vi "Helium Fridge Cool-Down-old.vi"() -> ()   [LabVIEW 2014]
uses:
  <vilib>/Analysis/8numeric.llb/1D Numeric Integration.vi
  <vilib>/express/express shared/transition.llb/Dynamic To Waveform Array.vi
  <vilib>/express/express signal manip/GetorSetDDTAttributes/Set DDT Attributes/SetT0.vi
  <vilib>/express/express shared/transition.llb/Waveform Array To Dynamic.vi
  <vilib>/express/express signal manip/GetorSetDDTAttributes/Set DDT Attributes/Set DDT Properties.xnode
  <vilib>/Analysis/NI_AALPro.lvlib
panel:
  out "?":dbl
  out "?":dbl
  out "?":dbl
  out "?":dbl
  out "Baseline X":dbl[](array[numeric])
  out "Session Out 2":refnum<visa-resource-name>
  out "error out 2":errorcluster {"code" format="%.0x"}
  out "token":dbl
  in  "error in 2":errorcluster {"code" format="%.0x"}
  in  "Session In 2":refnum<visa-resource-name>="HPSIGGEN"
  in  "Depth/Div Submit":bool
  out "Depth/Div (kHz)":dbl
  in  "Cent. Frq. Submit":bool
  out "Session Out":refnum<visa-resource-name>
  out "error out":errorcluster {"code" format="%.0x"}
  out "Central Frequency":dbl
  in  "error in":errorcluster {"code" format="%.0x"}
  in  "Session In":refnum<visa-resource-name>="HPSIGGEN"
  out "Cent. Freq. (MHz)":dbl
  out "Temp 2":bool
  out "Temperature Strip Chart":dynamicdata(graph)
  in  "TC Points/Measurement":dbl=20.0
  out "NMR":bool
  out "NMR Temp Error":bool
  out "Q Meter Temp":dynamicdata(graph)
  out "Zeroed Array":dbl[](array[numeric])
  out "Fit X values":dbl[](array[numeric])
  in  "Left wing 2":dbl
  in  "Right wing 2":dbl
  in  "Right wing":dbl
  in  "Left wing":dbl
  out "Fit":dbl[](array[numeric])
  in  "Submit":bool
  out "Is Flashing":bool
  in  "Error Beat":bool
  in  "Clear":bool
  in  "Comment":string
  out "Heartbeat":bool
  out "Most Recent Error":string
  out "Baseline Subtracted Integral vs. Time":dbl(graph)
  out "Time of Last Baseline":string
  out "Baseline Y":dbl[](array[numeric])
  in  "Baseline Subtract":bool
  in  "Get Baseline":bool
  out "Recording":bool
  out "Time of Last Recording":string
  in  "Record \nNMR Sweeps":bool
  in  "Depth/Div\n(MHz)":dbl=0.5
  in  "Central Freq. \n(MHz)":dbl=12.996
  in  "stop (F)":bool caption="Triangle Wave"
  in  "Triangle Wave\nRate (Hz)":dbl=15.0
  out "Time Elapsed \nDuring Sweeps (s)":dbl
  out "Lab Time":string
  out "Most Recent Error (NMR)":string
  out "Last Sweep Start Time":string
  out "Most Recent Error (Temp)":string
  out "Last Measurement Taken":string
  out "VI Start Time":string
  in  "Time Between\nTemp Ponts (s)":dbl=5.0
  out "Temp":bool
  out "NMR":bool
  in  "stop":bool
  out "Input Triangle Wave":dynamicdata(graph)
  out "Modulator":dynamicdata(graph)
  out "NMR":cluster{"Y":dbl[], "Y":dbl[]}[](graph)
  in  "# of Sweeps":dbl=1.0
  out "Resistance Strip Chart":dynamicdata(graph)
  in  "Heartbeat":bool
  in  "Temp Strip Chart":bool
  out "Errors":bool
  in  "Silence Flashing":bool
  # "Signal Generator Logic -- DO NOT TOUCH!!"
  # "Initialization and Logic Controls -- DO NOT TOUCH!!"
  # "Caitlyn's Work"
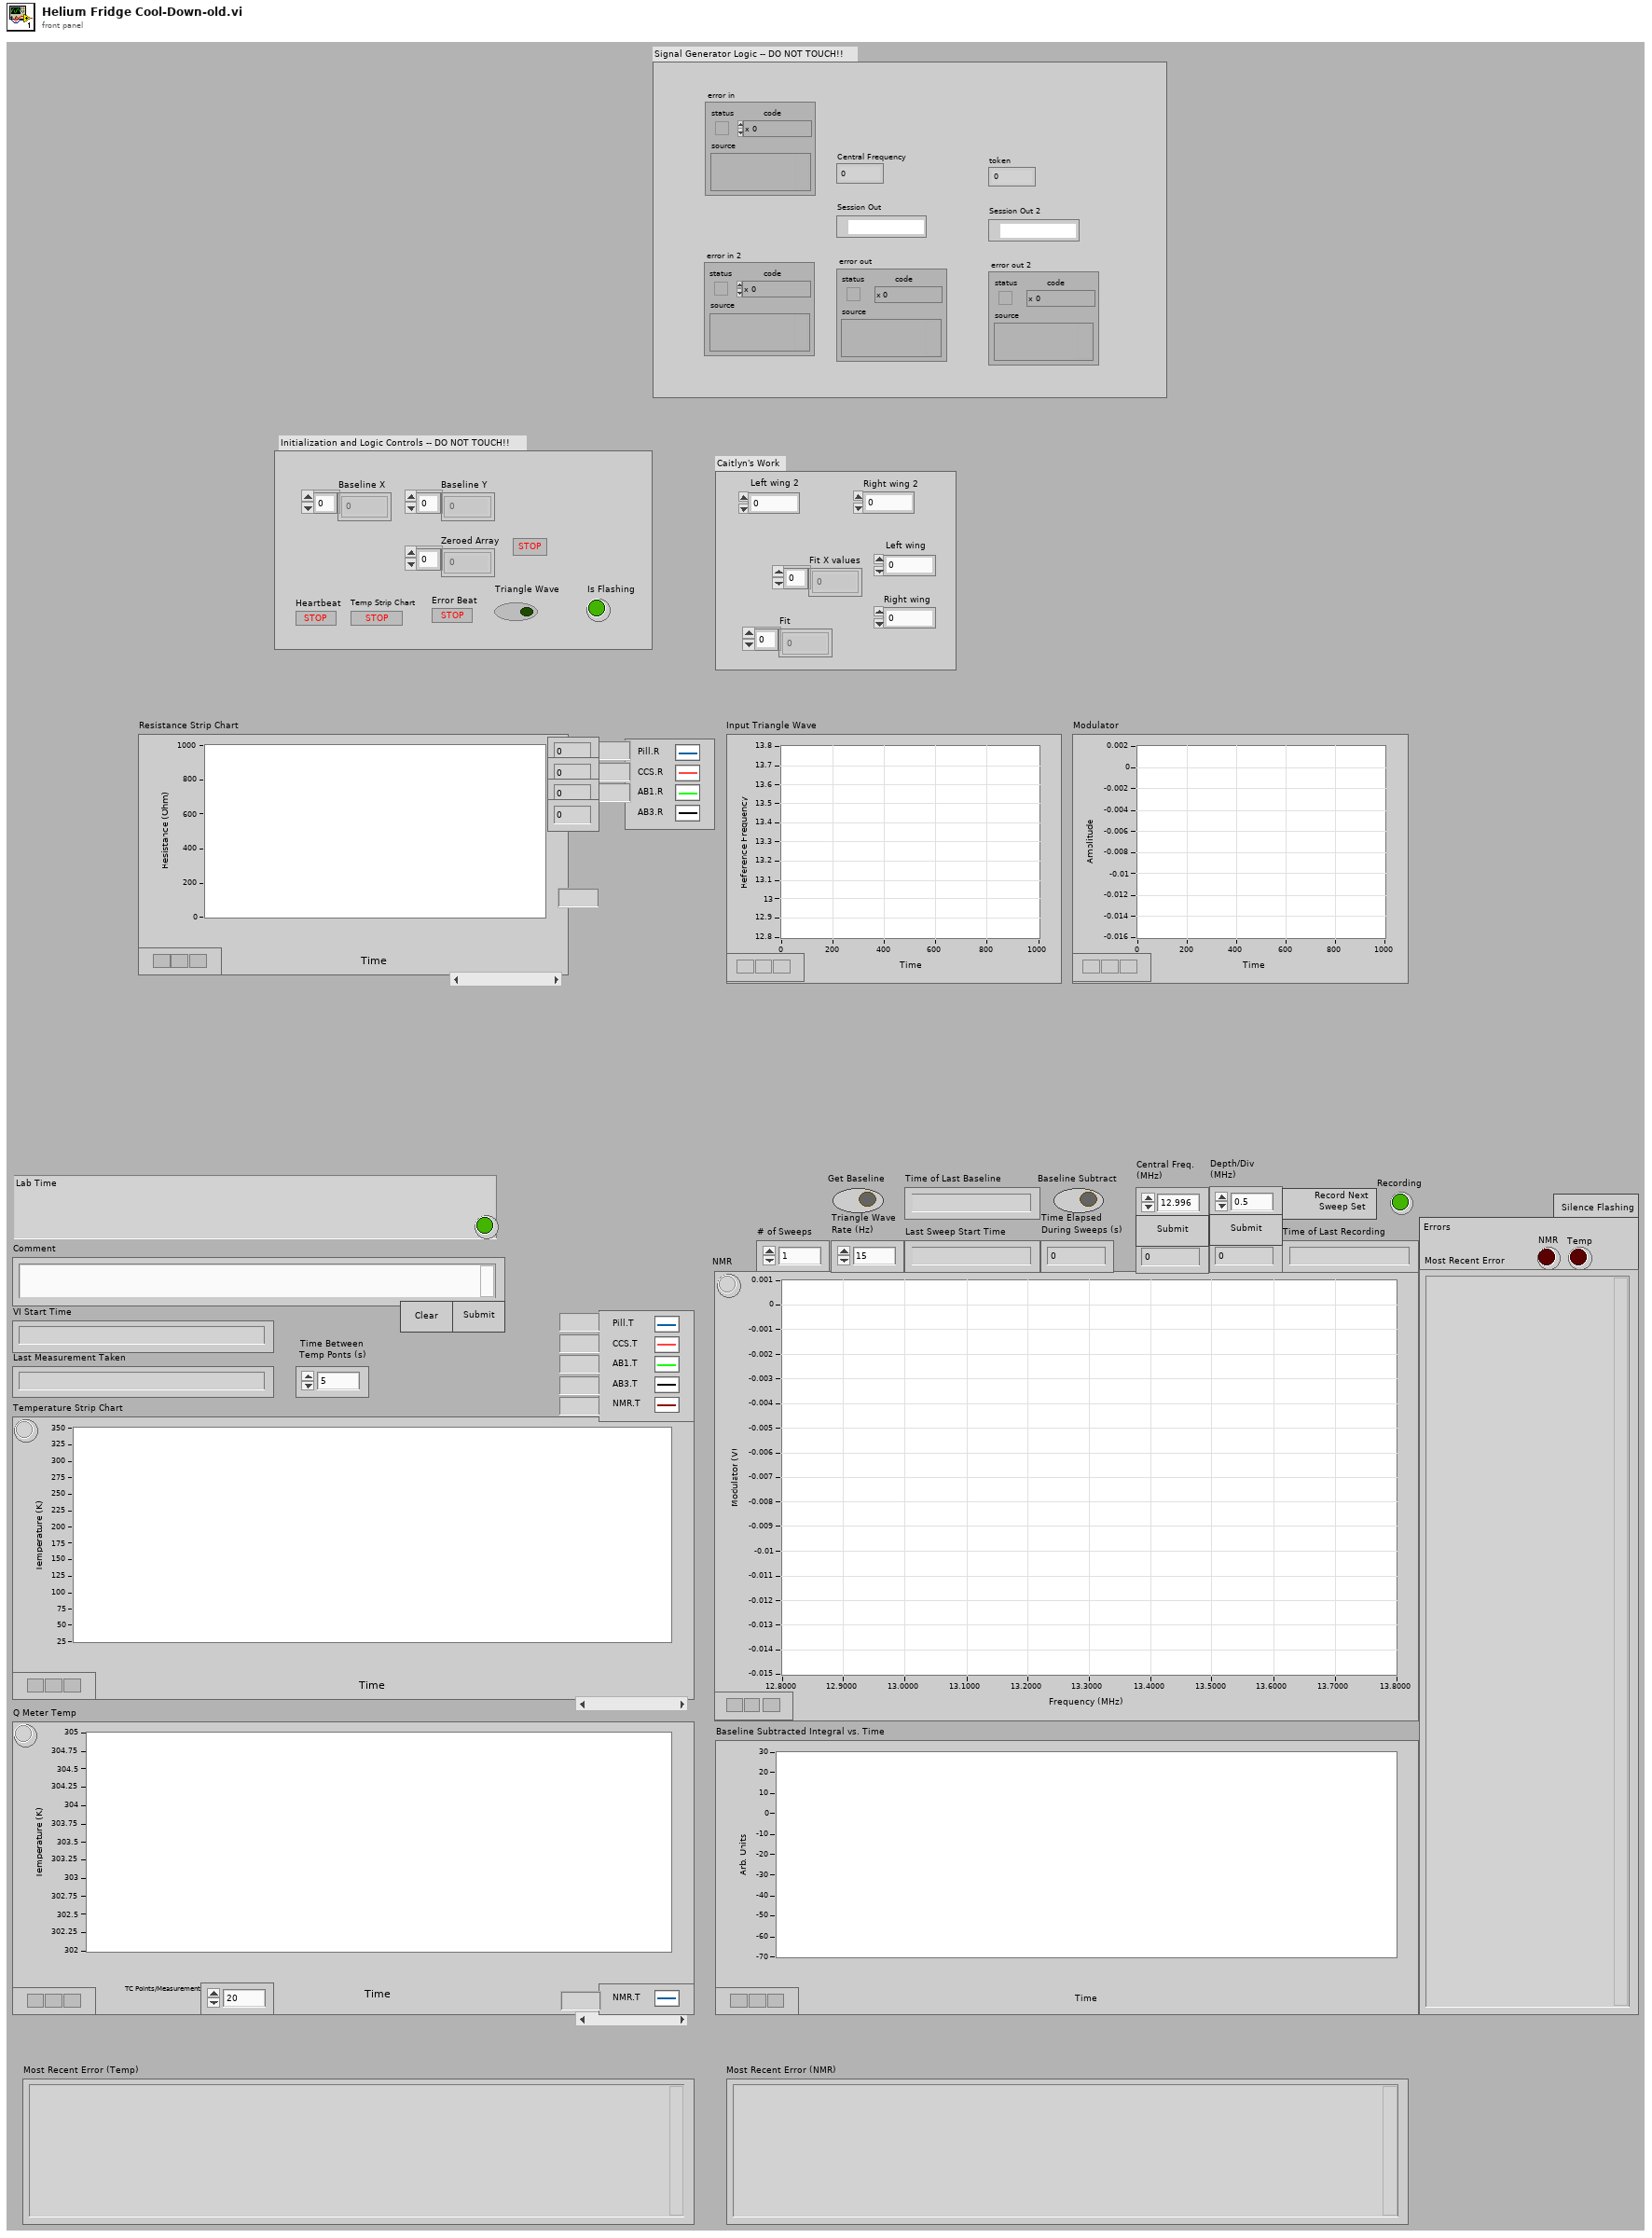
[diagram p1: front panel]
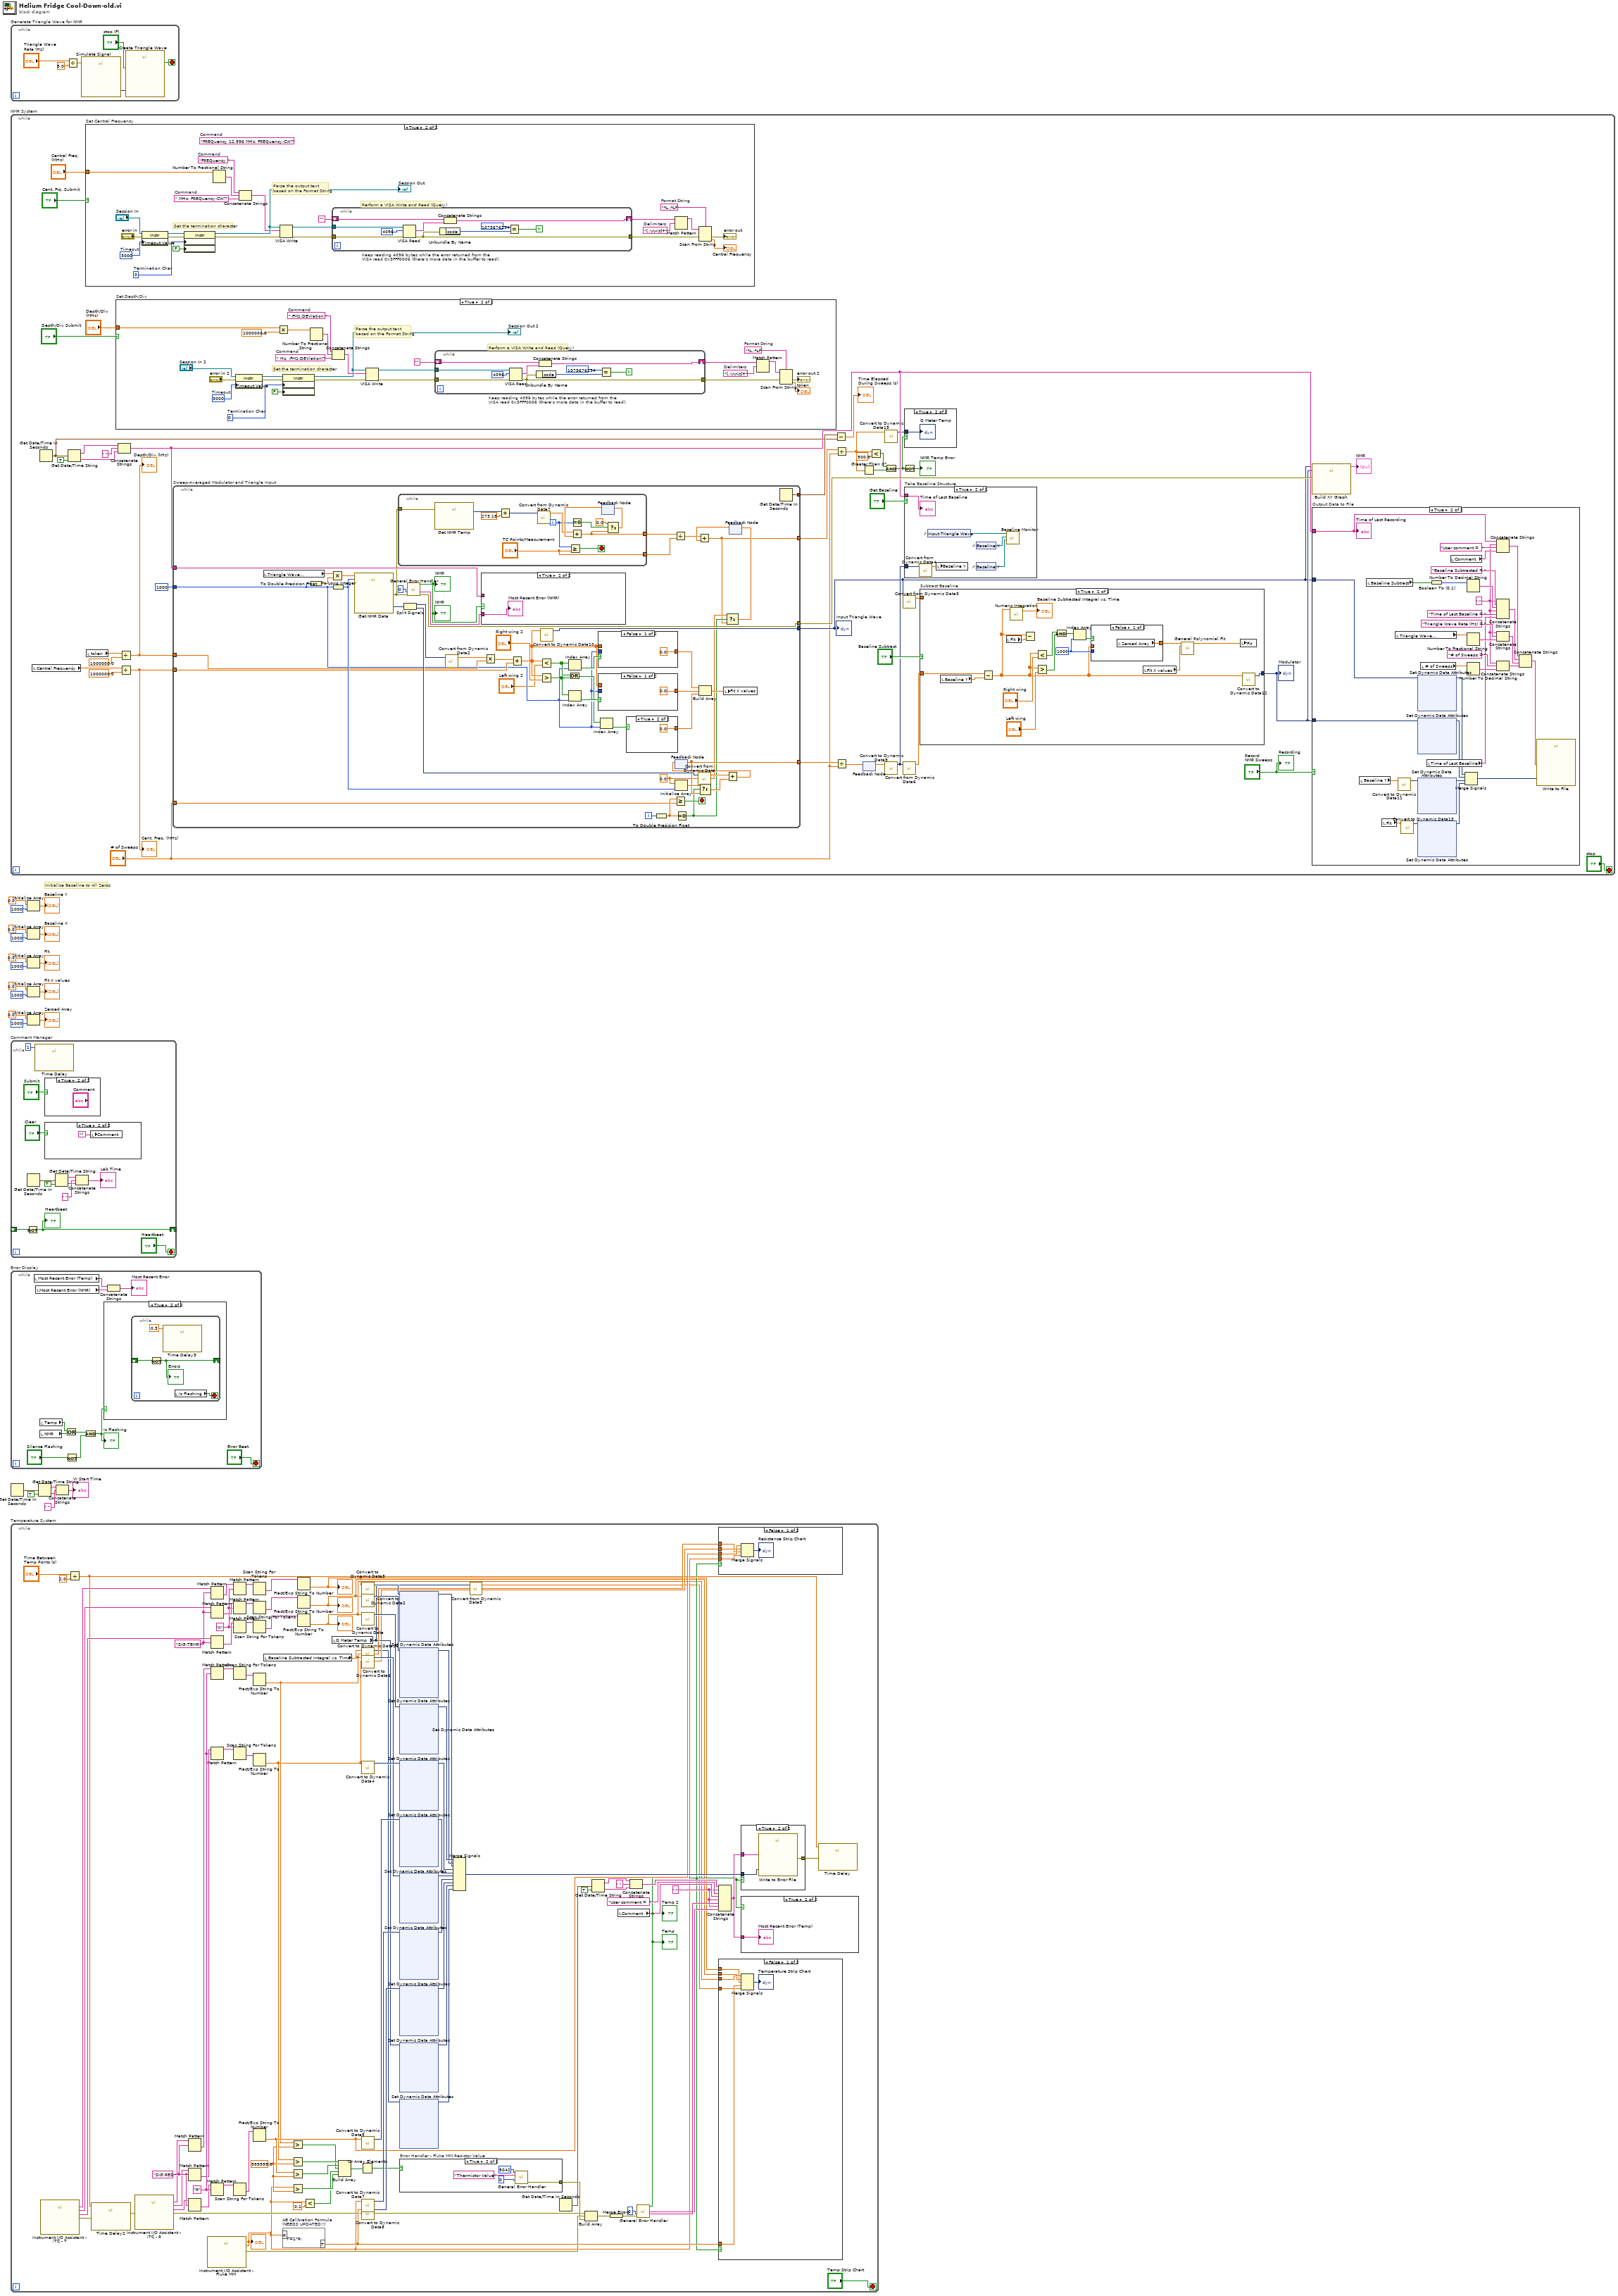
[diagram p0: block diagram]
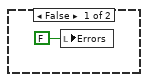
[diagram p2: hidden frame]
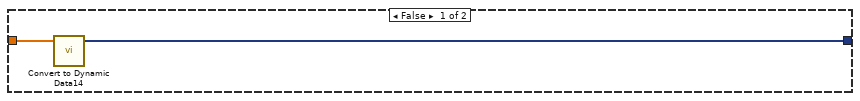
[diagram p6: hidden frame]
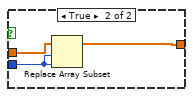
[diagram p7: hidden frame]
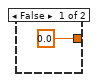
[diagram p10: hidden frame]
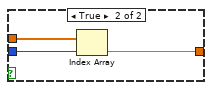
[diagram p11: hidden frame]
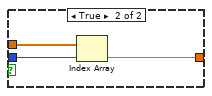
[diagram p12: hidden frame]
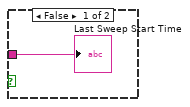
[diagram p13: hidden frame]
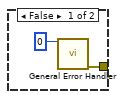
[diagram p16: hidden frame]
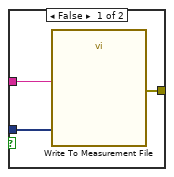
[diagram p19: hidden frame]
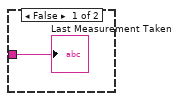
[diagram p20: hidden frame]
diagram:
  # "Initialize Baseline to All Zeros"
  n1 = while "Generate Triangle Wave for NMR" {
    stop <- w26 stop-if-true
    n2 = Divide(x="Triangle Wave\nRate (Hz)", y=5.0) -> (x/y=w22:dbl)
    n3 = call "Simulate Signal"("Frequency"=w22) -> ("Triangle"=w25:dynamicdata)  [unwired: 13 in, 1 out]
    n4 = call "Create Triangle Wave"("data"=w25, "stop (F)"="stop (F)") -> ("stopped"=w26:bool)  [unwired: 15 in, 2 out]
  }
  n5 = while "NMR System" {
    stop <- "stop" stop-if-true
    n6 = local read "Central Frequency"() -> (w34:dbl)
    n7 = Get Date/Time In Seconds() -> (seconds since 1Jan1904=w58:timestamp)
    n8 = Get Date/Time String(seconds (now)=w58, want seconds? (F)=TRUE) -> (date string=w61:string, time string=w63:string)  [unwired: 1 in]
    n9 = case "Set Central Frequency" shown="True" "Cent. Frq. Submit" {
      tunnel: "Central Freq. \n(MHz)" -> [_ w109]
      frame False {
      }
      frame True {
        w107 = " MHz; FREQuency:CW?"  # Command
        w110 = "FREQuency "  # Command
        w128 = "[,;\r\n\t]+"  # Delimiters
        w125 = "%.;%f"  # Format String
        (unwired) "FREQuency 12.996 MHz; FREQuency:CW?"  # Command
        w116 = u8 0  # Termination Char
        w111 = u32 3000  # Timeout
        # "Parse the output text based on the Format String"
        # "Perform a VISA Write and Read (Query)"
        # "Keep reading 4096 bytes while the error returned from the\nVISA read 0x3FFF0006 (there's more data in the buffer to read)."
        # "Set the termination character"
        n10 = property class="Instr"(reference="Session In", error in="error in", "General Settings:Timeout Value"=w111) -> (reference out=w117:refnum<visa-resource-name>, error out=w114:errorcluster)
        n11 = property class="Instr"(reference=w117, error in=w114, "Message Based Settings:Termination Character"=w116, "Message Based Settings:Termination Character Enable"=FALSE ("enable")) -> (reference out=w129:refnum<visa-resource-name>, error out=w115:errorcluster)
        "Session Out" <- w129
        n12 = Number To Fractional String(number=w109) -> (F-format string=w108:string)  [unwired: 3 in]
        n13 = Concatenate Strings(w110, w108, w107) -> (w106:string)
        n14 = VISA Write(VISA resource name=w129, write buffer=w106, error in (no error)=w115) -> (VISA resource name out=w119:refnum<visa-resource-name>, error out=w120:errorcluster)  [unwired: 1 out]
        n15 = while {
          tunnel: w119 -> [w136]
          shift-right: [w130] -> w123
          shift-left: "" -> [w135]
          tunnel: w120 -> [w133]
          tunnel: [w132] -> w121
          stop <- w131 continue-if-true
          n16 = VISA Read(VISA resource name=w136, byte count=u32 4096 ("byte count (0)"), error in (no error)=w133) -> (read buffer=w134:string, error out=w132:errorcluster)  [unwired: 2 out]
          n17 = Unbundle By Name(w132) -> ("code"=w138:i32)
          n18 = Concatenate Strings(w135, w134) -> (w130:string)
          n19 = Equal?(x=1073676294, y=w138) -> (x = y?=w131:bool)
        }
        n20 = Match Pattern(string=w123, regular expression=w128) -> (before substring=w124:string)  [unwired: 1 in, 3 out]
        n21 = Scan From String(format string=w125, input string=w124, error in=w121) -> (error out=→"error out":errorcluster, output 1=→"Central Frequency":dbl)  [unwired: 2 in, 2 out]
      }
    }
    n22 = local read "token"() -> (w29:dbl)
    n23 = case "Set Depth/Div" shown="True" "Depth/Div Submit" {
      tunnel: "Depth/Div\n(MHz)" -> [_ w71]
      frame False {
      }
      frame True {
        w73 = " Hz; :FM1:DEViation?"  # Command
        w78 = "[,;\r\n\t]+"  # Delimiters
        w81 = "%.;%f"  # Format String
        w75 = ":FM1:DEViation "  # Command
        w90 = u8 0  # Termination Char
        w95 = u32 3000  # Timeout
        # "Parse the output text based on the Format String"
        # "Perform a VISA Write and Read (Query)"
        # "Keep reading 4096 bytes while the error returned from the\nVISA read 0x3FFF0006 (there's more data in the buffer to read)."
        # "Set the termination character"
        n24 = property class="Instr"(reference="Session In 2", error in="error in 2", "General Settings:Timeout Value"=w95) -> (reference out=w89:refnum<visa-resource-name>, error out=w92:errorcluster)
        n25 = Multiply(x=w71, y=1000000.0) -> (x*y=w70:dbl)
        n26 = property class="Instr"(reference=w89, error in=w92, "Message Based Settings:Termination Character"=w90, "Message Based Settings:Termination Character Enable"=FALSE ("enable")) -> (reference out=w77:refnum<visa-resource-name>, error out=w91:errorcluster)
        "Session Out 2" <- w77
        n27 = Number To Fractional String(number=w70) -> (F-format string=w74:string)  [unwired: 3 in]
        n28 = Concatenate Strings(w75, w74, w73) -> (w76:string)
        n29 = VISA Write(VISA resource name=w77, write buffer=w76, error in (no error)=w91) -> (VISA resource name out=w87:refnum<visa-resource-name>, error out=w86:errorcluster)  [unwired: 1 out]
        n30 = while {
          tunnel: w87 -> [w102]
          shift-right: [w96] -> w83
          shift-left: "" -> [w101]
          tunnel: w86 -> [w99]
          tunnel: [w98] -> w85
          stop <- w97 continue-if-true
          n31 = VISA Read(VISA resource name=w102, byte count=u32 4096 ("byte count (0)"), error in (no error)=w99) -> (read buffer=w100:string, error out=w98:errorcluster)  [unwired: 2 out]
          n32 = Unbundle By Name(w98) -> ("code"=w104:i32)
          n33 = Concatenate Strings(w101, w100) -> (w96:string)
          n34 = Equal?(x=1073676294, y=w104) -> (x = y?=w97:bool)
        }
        n35 = Match Pattern(string=w83, regular expression=w78) -> (before substring=w82:string)  [unwired: 1 in, 3 out]
        n36 = Scan From String(format string=w81, input string=w82, error in=w85) -> (error out=→"error out 2":errorcluster, output 1=→"token":dbl)  [unwired: 2 in, 2 out]
      }
    }
    n37 = Concatenate Strings(w61, " ", w63) -> (w49:string)
    n38 = Divide(x=w29, y=1000000.0) -> (x/y=w28:dbl)
    "Depth/Div (kHz)" <- w28
    n39 = Divide(x=w34, y=1000000.0) -> (x/y=w32:dbl)
    "Cent. Freq. (MHz)" <- w32
    n40 = while "Sweep-Averaged Modulator and Triangle Input" {
      tunnel: "# of Sweeps" -> [w297]
      tunnel: 1000 -> [w288]
      tunnel: [w314] -> w66
      tunnel: w49 -> [w310]
      tunnel: [w309] -> w59
      tunnel: [w307] -> w56
      tunnel: w28 -> [w301]
      tunnel: w32 -> [w299]
      tunnel: [w298] -> w48
      tunnel: [w278] -> w37
      i -> [w320]
      stop <- w313 stop-if-true
      w281 = 0.0
      n41 = local read "Triangle Wave\nRate (Hz)"() -> (w306:dbl)
      n42 = To Double Precision Float(number=w288) -> (double precision float=w304:dbl)
      n43 = Multiply(x=w306, y=w304) -> (x*y=w308:dbl)
      n44 = To Long Integer(number=w288) -> (32bit integer=w305:i32)
      n45 = call "Get NMR Data"("rate"=w308, "number of samples"=w305) -> ("data"=w322:dynamicdata, "error out"=w273:errorcluster)  [unwired: 15 in, 1 out]
      n46 = while {
        tunnel: ["TC Points/Measurement"] -> w276
        tunnel: [w327] -> w275
        tunnel: w273 -> [w326]
        i -> [w325]
        stop <- w324 stop-if-true
        n47 = call "Get NMR Temp"("error in"=w326) -> ("data"=w329:dynamicdata)  [unwired: 16 in, 2 out]
        n48 = Add(x=w329, y=273.15) -> (x+y=w328:dynamicdata)
        n49 = call "Convert from Dynamic Data7"("Dynamic Data Type"=w328) -> ("Scalar"=w331:dbl)  [unwired: 3 in]
        n50 = Greater Or Equal?(x=w325, y="TC Points/Measurement") -> (x >= y?=w324:bool)
        n51 = Equal To 0?(x=w325) -> (x = 0?=w332:bool)
        n52 = feedback #1() -> (w334:dbl)  [unwired: 1 in]
        n53 = Add(x=w331, y=w334) -> (x+y=w327:dbl)
        n54 = Select(t=0.0, s=w332, f=w327) -> (s? t:f=w333:dbl)
        n55 = feedback-in #1(w333) -> ()
      }
      n56 = Split Signals(w322) -> (w303:dynamicdata, w321:dynamicdata)  [unwired: 2 in]
      n57 = call <vilib>:"General Error Handler.vi"("type of dialog (OK msg:1)"=0, "error in (no error)"=w273) -> ("error?"=w277:bool, "message"=w312:string, "error out"=w307:errorcluster)  [unwired: 9 in, 2 out]
      "NMR" <- w277
      "NMR" <- w277
      n58 = call "Convert from Dynamic Data2"("Dynamic Data Type"=w303) -> ("Array"=w302:dbl[])  [unwired: 3 in]
      n59 = case shown="True" w277 {
        tunnel: w312 -> [_ w347]
        tunnel: w310 -> [w346 _]
        frame False {
          "Last Sweep Start Time" <- w346
        }
        frame True {
          "Most Recent Error (NMR)" <- w347
        }
      }
      n60 = Multiply(x=w302, y=w301) -> (x*y=w300:dbl[])
      n61 = Add(x=w300, y=w299) -> (x+y=w294:dbl[])
      n62 = Less?(x=w294, y="Left wing 2") -> (x < y?=w290:bool[])
      n63 = Greater?(x=w294, y="Right wing 2") -> (0:w291:bool[])
      n64 = call "Convert to Dynamic Data10"("Array"=w294) -> ("Dynamic Data Type"=w298:dynamicdata)  [unwired: 3 in]
      n65 = Or(x=w290, y=w291) -> (x .or. y?=w289:bool[])
      n66 = Index Array(array=w290, index=w288) -> (element=w296:bool)
      n67 = Index Array(array=w291, index=w288) -> (element=w295:bool)
      n68 = case shown="False" w296 {
        tunnel: w294 -> [_ w345]
        tunnel: w288 -> [_ w344]
        tunnel: [0.0 w343] -> w292
        frame False {
        }
        frame True {
          n69 = Index Array(array=w345, index=w344) -> (element=w343:dbl)
        }
      }
      n70 = case shown="False" w295 {
        tunnel: w294 -> [_ w341]
        tunnel: w288 -> [_ w340]
        tunnel: [0.0 w339] -> w293
        frame False {
        }
        frame True {
          n71 = Index Array(array=w341, index=w340) -> (element=w339:dbl)
        }
      }
      n72 = Index Array(array=w289, index=w288) -> (element=w287:bool)
      n73 = case shown="True" w287 {
        tunnel: [0.0 0.0] -> w286
        frame False {
        }
        frame True {
        }
      }
      n74 = To Double Precision Float(number=w320) -> (double precision float=w319:dbl)
      n75 = Divide(x=w275, y=w276) -> (x/y=w274:dbl)
      n76 = Greater Or Equal?(x=w319, y=w297) -> (x >= y?=w313:bool)
      n77 = feedback #2() -> (w314:dbl[])  [unwired: 1 in]
      n78 = Initialize Array(w281, w305) -> (w317:dbl[])
      n79 = Equal To 0?(x=w319) -> (x = 0?=w282:bool)
      n80 = call "Convert from Dynamic Data"("Dynamic Data Type"=w321) -> ("Array"=w316:dbl[])  [unwired: 3 in]
      n81 = Build Array(w292, w293, w286) -> (w283:dbl[])
      n82 = Select(t=w317, s=w282, f=w314) -> (s? t:f=w318:dbl[])
      n83 = local write "Fit X values"(w283) -> ()
      n84 = Add(x=w316, y=w318) -> (x+y=w315:dbl[])
      n85 = feedback-in #2(w315) -> ()
      n86 = feedback #3() -> (w279:dbl)  [unwired: 1 in]
      n87 = Add(x=w274, y=w279) -> (x+y=w278:dbl)
      n88 = Select(t=w281, s=w282, f=w278) -> (s? t:f=w280:dbl)
      n89 = feedback-in #3(w280) -> ()
      n90 = Get Date/Time In Seconds() -> (seconds since 1Jan1904=w309:timestamp)
    }
    "Input Triangle Wave" <- w48
    n91 = Subtract(x=w59, y=w58) -> (x-y=→"Time Elapsed \nDuring Sweeps (s)":dbl)
    n92 = Divide(x=w37, y="# of Sweeps") -> (x/y=w38:dbl)
    n93 = Divide(x=w66, y="# of Sweeps") -> (x/y=w65:dbl[])
    n94 = Greater Than 0?(x=w38) -> (x > 0?=w45:bool)
    n95 = feedback-in #4(w65) -> ()
    n96 = feedback #4() -> (w64:dbl[])  [unwired: 1 in]
    n97 = Less?(x=w38, y=500.0) -> (x < y?=w42:bool)
    n98 = call "Convert to Dynamic Data15"("Double"=w38) -> ("Dynamic Data Type"=w40:dynamicdata)  [unwired: 3 in]
    n99 = And(x=w42, y=w45) -> (x .and. y?=w44:bool)
    n100 = call "Convert to Dynamic Data9"("Array"=w64) -> ("Dynamic Data Type"=w51:dynamicdata)  [unwired: 3 in]
    n101 = Not(x=w44) -> (.not. x?=→"NMR Temp Error":bool)
    n102 = call "Convert from Dynamic Data3"("Dynamic Data Type"=w48) -> ("Array"=w47:dbl[])  [unwired: 3 in]
    n103 = call "Convert from Dynamic Data6"("Dynamic Data Type"=w51) -> ("Array"=w46:dbl[])  [unwired: 3 in]
    n104 = case shown="True" w44 {
      tunnel: w40 -> [_ w140]
      frame False {
      }
      frame True {
        "Q Meter Temp" <- w140
      }
    }
    n105 = case "Take Baseline Structure" shown="True" "Get Baseline" {
      tunnel: w51 -> [_ w166]
      tunnel: w49 -> [_ w167]
      frame False {
      }
      frame True {
        n106 = call "Convert from Dynamic Data4"("Dynamic Data Type"=w166) -> ("Array"=w168:dbl[])  [unwired: 3 in]
        n107 = control-ref of="Input Triangle Wave"() -> (w165:refnum<vi>)
        n108 = local write "Baseline Y"(w168) -> ()
        n109 = control-ref of="Baseline X"() -> (w164:refnum<vi>)
        n110 = control-ref of="Baseline Y"() -> (w163:refnum<vi>)
        n111 = call "Baseline Monitor.vi"("reference 3"=w163, "reference in"=w164, "WaveformGraph in"=w165) -> ()  [unwired: 8 in, 1 out]
        "Time of Last Baseline" <- w167
      }
    }
    n112 = case "Subtract Baseline" shown="True" "Baseline Subtract" {
      tunnel: w46 -> [w142 w158]
      tunnel: [w141 w157] -> w50
      tunnel: w47 -> [_ _]
      frame False {
        n113 = call "Convert to Dynamic Data14"("Array"=w142) -> ("Dynamic Data Type"=w141:dynamicdata)  [unwired: 3 in]
      }
      frame True {
        w147 = 1000
        n114 = local read "Baseline Y"() -> (w155:dbl[])
        n115 = Subtract(x=w158, y=w155) -> (x-y=w143:dbl[])
        n116 = local read "Fit"() -> (w154:dbl[])
        n117 = call-poly <vilib>:"Numeric Integration.vi"("Input Array"=w143) -> ("result"=→"Baseline Subtracted Integral vs. Time":dbl)  [unwired: 2 in, 1 out]
        n118 = Subtract(x=w143, y=w154) -> ()  [unwired: 1 out]
        n119 = Less?(x=w143, y="Right wing") -> (x < y?=w151:bool[])
        n120 = Greater?(x=w143, y="Left wing") -> (0:w150:bool[])
        n121 = And(x=w151, y=w150) -> (x .and. y?=w149:bool[])
        n122 = Index Array(array=w149, index=w147) -> (element=w148:bool)
        n123 = case shown="False" w148 {
          tunnel: w143 -> [_ w162]
          tunnel: w147 -> [_ w160]
          tunnel: [w159 w161] -> w146
          frame False {
            n124 = local read "Zeroed Array"() -> (w159:dbl[])
          }
          frame True {
            n125 = Replace Array Subset(array=w162, new element=w160, index=w160) -> (w161:dbl[])
          }
        }
        n126 = local read "Fit X values"() -> (w144:dbl[])
        n127 = call <vilib>:"General Polynomial Fit.vi"("Y"=w146, "X"=w144) -> ("Best Polynomial Fit"=w145:dbl[])  [unwired: 10 in, 3 out]
        n128 = local write "Fit"(w145) -> ()
        n129 = call "Convert to Dynamic Data12"("Array"=w143) -> ("Dynamic Data Type"=w157:dynamicdata)  [unwired: 3 in]
      }
    }
    "Modulator" <- w50
    n130 = call "Build XY Graph"("error in (no error)"=w56, "Y Input"=w50, "X Input"=w48) -> ("XY Graph"=→"NMR":cluster{"Y":dbl[], "Y":dbl[]}[])  [unwired: 7 in, 1 out]
    n131 = case "Output Data to File" shown="True" "Record \nNMR Sweeps" {
      tunnel: w49 -> [_ w189]
      tunnel: w50 -> [_ w196]
      tunnel: w48 -> [_ w195]
      frame False {
      }
      frame True {
        w173 = ";"
        n132 = local read "Baseline Y"() -> (w194:dbl[])
        n133 = local read "Baseline Subtract"() -> (w191:bool)
        n134 = local read "Fit"() -> (w172:dbl[])
        n135 = local read "Triangle Wave\nRate (Hz)"() -> (w192:dbl)
        n136 = call "Convert to Dynamic Data11"("Array"=w194) -> ("Dynamic Data Type"=w193:dynamicdata)  [unwired: 3 in]
        n137 = call "Convert to Dynamic Data13"("Array"=w172) -> ("Dynamic Data Type"=w171:dynamicdata)  [unwired: 3 in]
        n138 = xnode "Set Dynamic Data Attributes"("Signals In"=w195) -> ("Signals Out"=w200:dynamicdata)  [unwired: 4 in, 1 out]
        n139 = xnode "Set Dynamic Data Attributes"("Signals In"=w196) -> ("Signals Out"=w198:dynamicdata)  [unwired: 4 in, 1 out]
        n140 = xnode "Set Dynamic Data Attributes"("Signals In"=w193) -> ("Signals Out"=w170:dynamicdata)  [unwired: 4 in, 1 out]
        n141 = xnode "Set Dynamic Data Attributes"("Signals In"=w171) -> ("Signals Out"=w169:dynamicdata)  [unwired: 4 in, 1 out]
        n142 = local read "# of Sweeps"() -> (w197:dbl)
        n143 = local read "Time of Last Baseline"() -> (w178:string)
        n144 = Boolean To (0,1)(Boolean=w191) -> (0, 1=w190:i16)
        n145 = local read "Comment"() -> (w187:string)
        n146 = Merge Signals(w200, w198, w170, w169) -> (w199:dynamicdata)
        n147 = Number To Decimal String(number=w190) -> (decimal integer string=w183:string)  [unwired: 1 in]
        n148 = Number To Fractional String(number=w192) -> (F-format string=w181:string)  [unwired: 3 in]
        n149 = Number To Decimal String(number=w197) -> (decimal integer string=w185:string)  [unwired: 1 in]
        n150 = Concatenate Strings(w189, w173, "User comment =  ", w187) -> (w180:string)
        n151 = Concatenate Strings(w173, "Baseline Subtracted = ", w183, w173, "Time of Last Baseline = ", w178) -> (w177:string)
        n152 = Concatenate Strings(w173, "Triangle Wave Rate (Hz) = ", w181) -> (w176:string)
        n153 = Concatenate Strings(w173, "# of Sweeps = ", w185) -> (w175:string)
        n154 = Concatenate Strings(w180, w177, w176, w175) -> (w174:string)
        n155 = call "Write to File"("Signals"=w199, "Comment"=w174) -> ()  [unwired: 15 in, 3 out]
        "Time of Last Recording" <- w189
      }
    }
    "Recording" <- "Record \nNMR Sweeps"
  }
  n156 = while "Comment Manager" {
    shift-right: [w356] -> _
    shift-left: _ -> [w359]
    stop <- "Heartbeat" stop-if-true
    n157 = Not(x=w359) -> (.not. x?=w356:bool)
    "Heartbeat" <- w356
    n158 = Get Date/Time In Seconds() -> (seconds since 1Jan1904=w354:timestamp)
    n159 = call "Time Delay"("Delay Time (s)"=1) -> ()  [unwired: 10 in, 1 out]
    n160 = case shown="True" "Submit" {
      frame False {
      }
      frame True {
      }
    }
    n161 = case shown="True" "Clear" {
      frame False {
      }
      frame True {
        n162 = local write "Comment"("") -> ()
      }
    }
    n163 = Get Date/Time String(seconds (now)=w354, want seconds? (F)=TRUE) -> (date string=w353:string, time string=w351:string)  [unwired: 1 in]
    n164 = Concatenate Strings(w353, " ", w351) -> (→"Lab Time":string)
  }
  n165 = while "Error Display" {
    stop <- "Error Beat" stop-if-true
    n166 = local read "Most Recent Error (Temp)"() -> (w361:string)
    n167 = local read "Most Recent Error (NMR)"() -> (w362:string)
    n168 = local read "Temp"() -> (w370:bool)
    n169 = local read "NMR"() -> (w369:bool)
    n170 = Or(x=w370, y=w369) -> (x .or. y?=w367:bool)
    n171 = Not(x="Silence Flashing") -> (.not. x?=w365:bool)
    n172 = And(x=w367, y=w365) -> (x .and. y?=w364:bool)
    "Is Flashing" <- w364
    n173 = case shown="True" w364 {
      frame False {
        n174 = local write "Errors"(FALSE) -> ()
      }
      frame True {
        n175 = while {
          shift-right: [w373] -> _
          shift-left: _ -> [w375]
          stop <- w372 stop-if-true
          n176 = Not(x=w375) -> (.not. x?=w373:bool)
          "Errors" <- w373
          n177 = call "Time Delay3"("Delay Time (s)"=0.3) -> ()  [unwired: 10 in, 1 out]
          n178 = local read "Is Flashing"() -> (w372:bool)
        }
      }
    }
    n179 = Concatenate Strings(w361, w362) -> (→"Most Recent Error":string)
  }
  n180 = Get Date/Time In Seconds() -> (seconds since 1Jan1904=w20:timestamp)
  n181 = while "Temperature System" {
    stop <- "Temp Strip Chart" stop-if-true
    w389 = ";"
    w410 = 999999.0
    w439 = "R"
    w440 = "SIG:RES:"
    w446 = "SIG:TEMP:"
    w445 = "K"
    n182 = call "Instrument I/O Assistant - iTC - T"() -> ("AB1.T"=w444:string, "CCS.T"=w449:string, "Pill.T"=w452:string, "error out"=w402:errorcluster)  [unwired: 23 in, 1 out]
    n183 = Divide(x="Time Between\nTemp Ponts (s)", y=2.0) -> (x/y=w397:dbl)
    n184 = call "Time Delay2"("error in (no error)"=w402, "Delay Time (s)"=w397) -> ("error out"=w403:errorcluster)  [unwired: 9 in]
    n185 = call "Instrument I/O Assistant - iTC - R"("error in"=w403) -> ("AB1.R"=w399:string, "CCS.R"=w400:string, "Pill.R"=w401:string, "error out"=w404:errorcluster)  [unwired: 22 in, 1 out]
    n186 = Match Pattern(string=w399, regular expression=w440) -> (after substring=w436:string)  [unwired: 1 in, 3 out]
    n187 = Match Pattern(string=w400, regular expression=w440) -> (after substring=w438:string)  [unwired: 1 in, 3 out]
    n188 = Match Pattern(string=w401, regular expression=w440) -> (after substring=w437:string)  [unwired: 1 in, 3 out]
    n189 = call "Instrument I/O Assistant - Fluke MM"() -> ("AB3.R"=w379:dbl, "error out"=w407:errorcluster)  [unwired: 25 in, 1 out]
    "?" <- w379
    n190 = Match Pattern(string=w444, regular expression=w446) -> (after substring=w443:string)  [unwired: 1 in, 3 out]
    n191 = Match Pattern(string=w449, regular expression=w446) -> (after substring=w448:string)  [unwired: 1 in, 3 out]
    n192 = Match Pattern(string=w452, regular expression=w446) -> (after substring=w451:string)  [unwired: 1 in, 3 out]
    n193 = Match Pattern(string=w436, regular expression=w439) -> (before substring=w433:string)  [unwired: 1 in, 3 out]
    n194 = Match Pattern(string=w438, regular expression=w439) -> (before substring=w435:string)  [unwired: 1 in, 3 out]
    n195 = Match Pattern(string=w437, regular expression=w439) -> (before substring=w434:string)  [unwired: 1 in, 3 out]
    n196 = Match Pattern(string=w443, regular expression=w445) -> (before substring=w442:string)  [unwired: 1 in, 3 out]
    n197 = Match Pattern(string=w448, regular expression=w445) -> (before substring=w447:string)  [unwired: 1 in, 3 out]
    n198 = Match Pattern(string=w451, regular expression=w445) -> (before substring=w450:string)  [unwired: 1 in, 3 out]
    n199 = Scan String For Tokens(9:w433) -> (1:w430:string)  [unwired: 5 in, 3 out]
    n200 = Scan String For Tokens(9:w435) -> (1:w432:string)  [unwired: 5 in, 3 out]
    n201 = Scan String For Tokens(9:w434) -> (1:w431:string)  [unwired: 5 in, 3 out]
    n202 = Scan String For Tokens(9:w442) -> (1:w466:string)  [unwired: 5 in, 3 out]
    n203 = Scan String For Tokens(9:w447) -> (1:w467:string)  [unwired: 5 in, 3 out]
    n204 = Scan String For Tokens(9:w450) -> (1:w469:string)  [unwired: 5 in, 3 out]
    n205 = Fract/Exp String To Number(string=w430) -> (number=w414:dbl)  [unwired: 3 in, 1 out]
    n206 = Fract/Exp String To Number(string=w432) -> (number=w383:dbl)  [unwired: 3 in, 1 out]
    n207 = Fract/Exp String To Number(string=w431) -> (number=w415:dbl)  [unwired: 3 in, 1 out]
    n208 = local read "Baseline Subtracted Integral vs. Time"() -> (w378:dbl)
    n209 = formula code="T=1*R;" "AB Calibration Formula\n(NEEDS UPDATED!!)"("R"=w379) -> ("T"=w420:dbl)
    n210 = Greater?(x=w414, y=w410) -> (0:w411:bool)
    n211 = Greater?(x=w383, y=w410) -> (0:w413:bool)
    n212 = Greater?(x=w415, y=w410) -> (0:w412:bool)
    n213 = Greater?(x=w379, y=w410) -> (0:w409:bool)
    n214 = Fract/Exp String To Number(string=w466) -> (number=w380:dbl)  [unwired: 3 in, 1 out]
    "?" <- w380
    n215 = Fract/Exp String To Number(string=w467) -> (number=w381:dbl)  [unwired: 3 in, 1 out]
    "?" <- w381
    n216 = Fract/Exp String To Number(string=w469) -> (number=w382:dbl)  [unwired: 3 in, 1 out]
    "?" <- w382
    n217 = Less?(x=w379, y=0.1) -> (x < y?=w408:bool)
    n218 = local read "Q Meter Temp"() -> (w385:dynamicdata)
    n219 = Build Array(w413, w412, w411, w408, w409) -> (w417:bool[])
    n220 = Or Array Elements(Boolean array=w417) -> (logical OR=w416:bool)
    n221 = call "Convert to Dynamic Data3"("Double"=w380) -> ("Dynamic Data Type"=w457:dynamicdata)  [unwired: 3 in]
    n222 = call "Convert to Dynamic Data2"("Double"=w381) -> ("Dynamic Data Type"=w458:dynamicdata)  [unwired: 3 in]
    n223 = call "Convert to Dynamic Data"("Double"=w382) -> ("Dynamic Data Type"=w460:dynamicdata)  [unwired: 3 in]
    n224 = call "Convert to Dynamic Data16"("Double"=w378) -> ("Dynamic Data Type"=w377:dynamicdata)  [unwired: 3 in]
    n225 = call "Convert to Dynamic Data6"("Double"=w414) -> ("Dynamic Data Type"=w427:dynamicdata)  [unwired: 3 in]
    n226 = call "Convert to Dynamic Data4"("Double"=w383) -> ("Dynamic Data Type"=w429:dynamicdata)  [unwired: 3 in]
    n227 = call "Convert to Dynamic Data5"("Double"=w415) -> ("Dynamic Data Type"=w428:dynamicdata)  [unwired: 3 in]
    n228 = call "Convert to Dynamic Data7"("Double"=w379) -> ("Dynamic Data Type"=w423:dynamicdata)  [unwired: 3 in]
    n229 = call "Convert to Dynamic Data8"("Double"=w420) -> ("Dynamic Data Type"=w419:dynamicdata)  [unwired: 3 in]
    n230 = xnode "Set Dynamic Data Attributes"("Signals In"=w457) -> ("Signals Out"=w455:dynamicdata)  [unwired: 4 in, 1 out]
    n231 = xnode "Set Dynamic Data Attributes"("Signals In"=w458) -> ("Signals Out"=w456:dynamicdata)  [unwired: 4 in, 1 out]
    n232 = xnode "Set Dynamic Data Attributes"("Signals In"=w460) -> ("Signals Out"=w459:dynamicdata)  [unwired: 4 in, 1 out]
    n233 = xnode "Set Dynamic Data Attributes"("Signals In"=w429) -> ("Signals Out"=w426:dynamicdata)  [unwired: 4 in, 1 out]
    n234 = xnode "Set Dynamic Data Attributes"("Signals In"=w428) -> ("Signals Out"=w425:dynamicdata)  [unwired: 4 in, 1 out]
    n235 = xnode "Set Dynamic Data Attributes"("Signals In"=w427) -> ("Signals Out"=w424:dynamicdata)  [unwired: 4 in, 1 out]
    n236 = xnode "Set Dynamic Data Attributes"("Signals In"=w423) -> ("Signals Out"=w422:dynamicdata)  [unwired: 4 in, 1 out]
    n237 = xnode "Set Dynamic Data Attributes"("Signals In"=w419) -> ("Signals Out"=w418:dynamicdata)  [unwired: 4 in, 1 out]
    n238 = xnode "Set Dynamic Data Attributes"("Signals In"=w385) -> ("Signals Out"=w388:dynamicdata)  [unwired: 4 in, 1 out]
    n239 = xnode "Set Dynamic Data Attributes"("Signals In"=w377) -> ("Signals Out"=w376:dynamicdata)  [unwired: 4 in, 1 out]
    n240 = case "Error Handler - Fluke MM Resistor Value" shown="True" w416 {
      tunnel: [w506 w511] -> w406
      frame False {
        n241 = call <vilib>:"General Error Handler.vi"("[error code] (0)"=0) -> ("error out"=w506:errorcluster)  [unwired: 10 in, 4 out]
      }
      frame True {
        n242 = call <vilib>:"General Error Handler.vi"("[error code] (0)"=5042, "[error source] (\" \")"="Thermistor Value", "type of dialog (OK msg:1)"=0) -> ("error out"=w511:errorcluster)  [unwired: 8 in, 4 out]
      }
    }
    n243 = Merge Signals(w459, w456, w455, w426, w425, w424, w422, w418, w388, w376) -> (w454:dynamicdata)
    n244 = call "Convert from Dynamic Data5"("Dynamic Data Type"=w385) -> ("Scalar"=w384:dbl)  [unwired: 3 in]
    n245 = Get Date/Time In Seconds() -> (seconds since 1Jan1904=w465:timestamp)
    n246 = Build Array(w404, w407, w406) -> (w405:errorcluster[])
    n247 = Get Date/Time String(seconds (now)=w465, want seconds? (F)=TRUE) -> (date string=w463:string, time string=w461:string)  [unwired: 1 in]
    n248 = Merge Errors(w405) -> (w421:errorcluster)
    n249 = local read "Comment"() -> (w394:string)
    n250 = Concatenate Strings(w463, " ", w461) -> (w390:string)
    n251 = call <vilib>:"General Error Handler.vi"("type of dialog (OK msg:1)"=0, "error in (no error)"=w421) -> ("error?"=w386:bool, "source out"=w391:string, "message"=w393:string)  [unwired: 9 in, 2 out]
    "Temp" <- w386
    "Temp 2" <- w386
    n252 = case shown="False" w386 {
      tunnel: w415 -> [w606 _]
      tunnel: w383 -> [w605 _]
      tunnel: w414 -> [w604 _]
      tunnel: w379 -> [w603 _]
      frame False {
        n253 = Merge Signals(w606, w605, w604, w603) -> (→"Resistance Strip Chart":dynamicdata)
      }
      frame True {
      }
    }
    n254 = Concatenate Strings(w390, w389, "User comment =  ", w394, w389, w393, w389, w391) -> (w392:string)
    n255 = case shown="False" w386 {
      tunnel: w382 -> [w612 _]
      tunnel: w381 -> [w611 _]
      tunnel: w380 -> [w610 _]
      tunnel: w420 -> [w609 _]
      tunnel: w384 -> [w607 _]
      frame False {
        n256 = Merge Signals(w612, w611, w610, w609, w607) -> (→"Temperature Strip Chart":dynamicdata)
      }
      frame True {
      }
    }
    n257 = case shown="True" w386 {
      tunnel: w454 -> [w615 w618]
      tunnel: w392 -> [w614 w617]
      tunnel: [w613 w616] -> w441
      frame False {
        n258 = call "Write To Measurement File"("Signals"=w615, "Comment"=w614) -> ("error out"=w613:errorcluster)  [unwired: 15 in, 2 out]
      }
      frame True {
        n259 = call "Write to Error File"("Signals"=w618, "Comment"=w617) -> ("error out"=w616:errorcluster)  [unwired: 15 in, 2 out]
      }
    }
    n260 = case shown="True" w386 {
      tunnel: w392 -> [w673 w674]
      frame False {
        "Last Measurement Taken" <- w673
      }
      frame True {
        "Most Recent Error (Temp)" <- w674
      }
    }
    n261 = call "Time Delay"("error in (no error)"=w441, "Delay Time (s)"=w397) -> ()  [unwired: 9 in, 1 out]
  }
  n262 = Initialize Array(0.0, 1000) -> (→"Baseline Y":dbl[])
  n263 = Initialize Array(0.0, 1000) -> (→"Baseline X":dbl[])
  n264 = Initialize Array(0.0 ("number"), 1000) -> (→"Fit":dbl[])
  n265 = Initialize Array(0.0, 1000) -> (→"Fit X values":dbl[])
  n266 = Initialize Array(0.0, 1000) -> (→"Zeroed Array":dbl[])
  n267 = Get Date/Time String(seconds (now)=w20, want seconds? (F)=TRUE) -> (date string=w19:string, time string=w17:string)  [unwired: 1 in]
  n268 = Concatenate Strings(w19, " ", w17) -> (→"VI Start Time":string)
